vi "SaveTrendData.vi"(6 "registry":T13, 8 "error in (no error)":errorcluster, 9 "data":T9, 10 "data event config":T17, 11 "data event":T1) -> (0 "error out":errorcluster, 3 "data event out":T1)   [LabVIEW 2017, in "DataEventCreator.lvlib"]
uses:
  <vilib>/addons/InsightCM/Devices/Shared/Common/DataEventCreator/DataEventCreator.lvlib
  <vilib>/addons/InsightCM/Devices/Shared/Cms/CmsDataEventCreator/controls/DataEventConfig.ctl
  <vilib>/addons/InsightCM/Devices/Shared/Cms/CmsDataEventCreator/controls/AcqParams.ctl
  <vilib>/addons/InsightCM/Devices/Shared/Common/DataAccumulator/controls/AccumulationSettings.ctl
  <vilib>/addons/InsightCM/Devices/Shared/Common/DataAccumulator/controls/accumulationType.ctl
  <vilib>/addons/InsightCM/Devices/Shared/Common/DVRBuffer/controls/BufferLocation.ctl
  <vilib>/addons/PointValueMap/controls/PointMap.ctl
  <vilib>/addons/InsightCM/Devices/Shared/Cms/CmsDataEventCreator/controls/GroupRegistry.ctl
  <vilib>/addons/InsightCM/Devices/Shared/Cms/CmsDataEventCreator/controls/DataSetRegistry.ctl
  <vilib>/addons/InsightCM/Devices/Shared/Common/DataEvent/controls/DataSetType.ctl
  <vilib>/addons/InsightCM/Devices/Shared/Common/DataEventCreator/controls/Registry_Trend.ctl
  <vilib>/addons/InsightCM/Devices/Shared/Common/DataFlow/controls/Data.ctl
  <vilib>/addons/InsightCM/Utilities/DataAccessors/controls/wfmSGL_DVR.ctl
  <vilib>/addons/InsightCM/Devices/Shared/Common/DataFlow/controls/Type.ctl
  <vilib>/addons/InsightCM/Devices/Shared/Common/DataEvent/controls/Event.ctl
  <vilib>/addons/InsightCM/MessageBus/Base/controls/DataEvent.ctl
  <vilib>/addons/InsightCM/MessageBus/Base/controls/KeyValuePair.ctl
  <vilib>/addons/InsightCM/Devices/Shared/Common/DataEvent/controls/DataSet.ctl
  <vilib>/addons/InsightCM/MessageBus/Base/controls/DataSetMetadata.ctl
  <vilib>/addons/InsightCM/MessageBus/Base/controls/TrendPoint.ctl
  <vilib>/addons/InsightCM/MessageBus/Base/controls/TrendAlarmUpdate.ctl
  <vilib>/addons/InsightCM/MessageBus/Base/controls/TrendAlarmTransition.ctl
  <vilib>/addons/PointValueMap/subVIs/Point_Read_double.vi
  <vilib>/addons/PointValueMap/PointValueMap.lvlib
  <vilib>/addons/InsightCM/Devices/Shared/Common/DataFlow/DataFlow.lvlib
  <vilib>/addons/InsightCM/Devices/Shared/Common/DataEvent/DataEvent.lvlib
  <vilib>/addons/InsightCM/Devices/Shared/Cms/CmsDataEventCreator/CmsDataEventCreator.lvlib
  <vilib>/addons/InsightCM/Devices/Shared/Common/DataAccumulator/DataAccumulator.lvlib
  <vilib>/addons/InsightCM/Devices/Shared/Common/DVRBuffer/DVRBuffer.lvlib
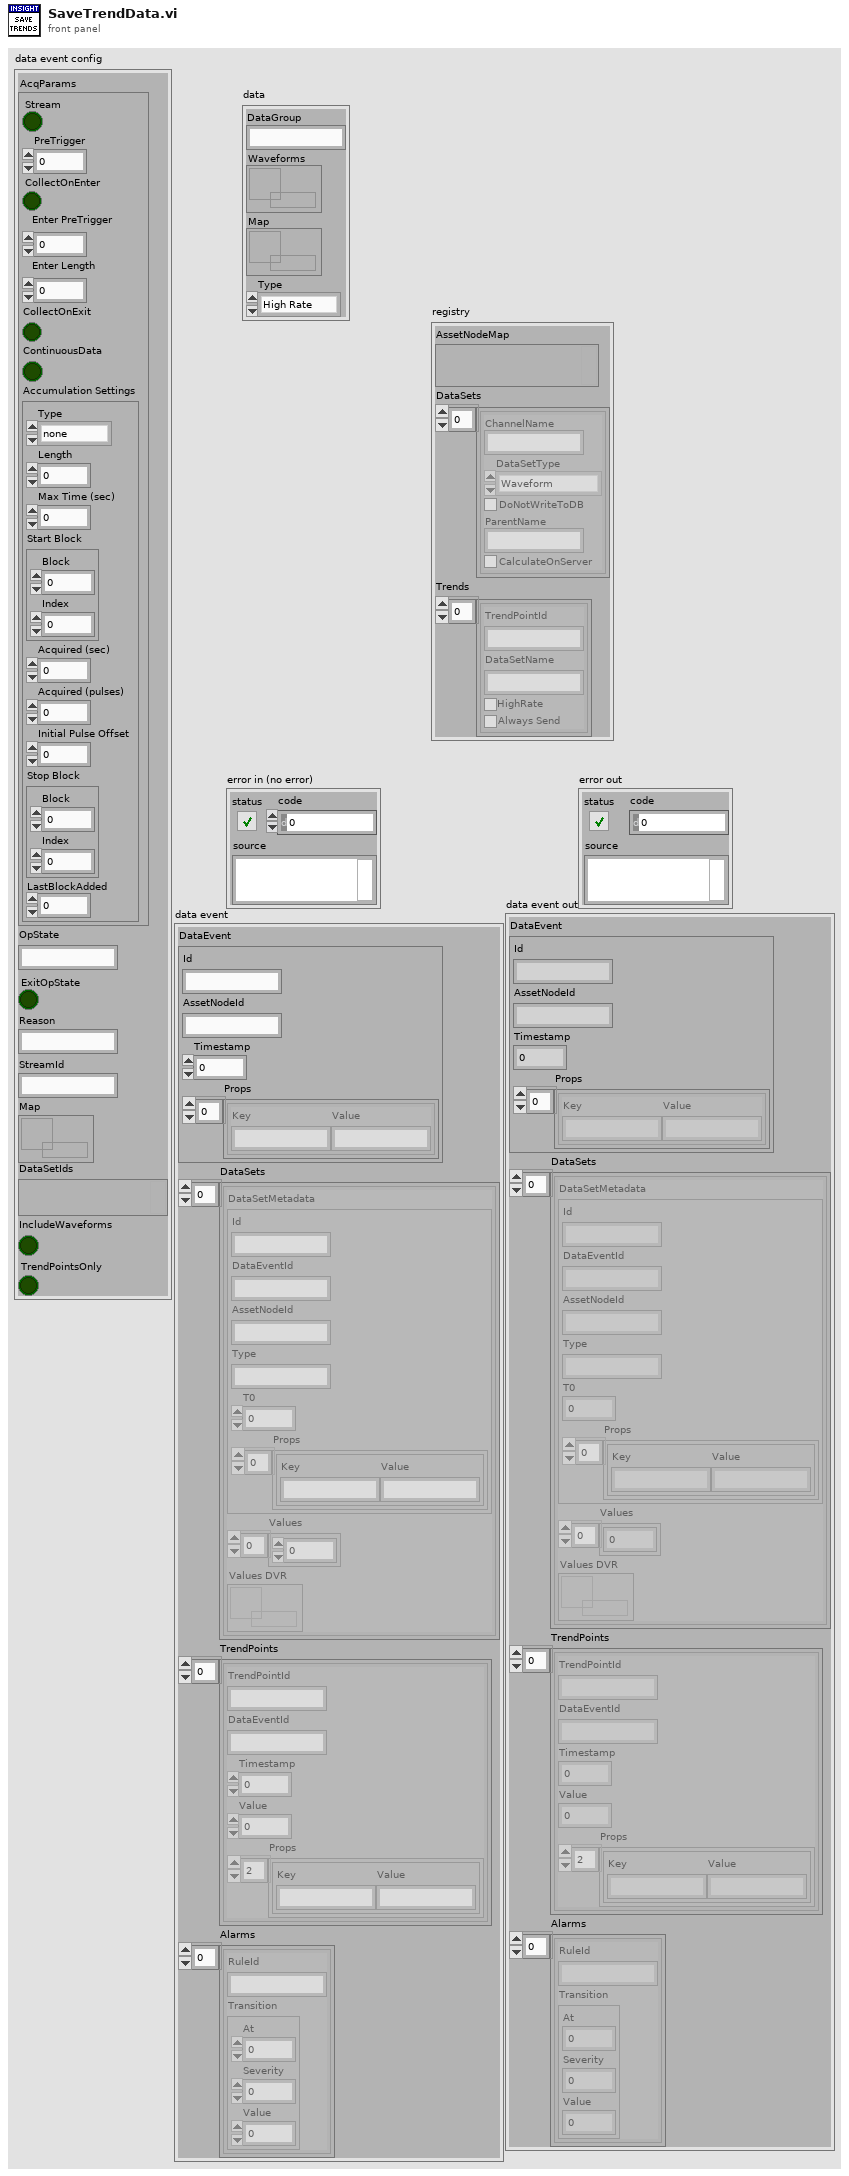
[diagram p1: front panel]
types:
  T1 = typedef "DataEvent.lvlib/Event.ctl" = cluster{"DataEvent":T2, "DataSets":T4[], "TrendPoints":T6[], "Alarms":T7[]}
  T2 = typedef "DataEvent.ctl" = cluster{"Id":string, "AssetNodeId":string, "Timestamp":i64, "Props":T3[]}
  T3 = typedef "KeyValuePair.ctl" = cluster{"Key":string, "Value":string}
  T4 = typedef "DataEvent.lvlib/DataSet.ctl" = cluster{"DataSetMetadata":T5, "Values":sgl[], "Values DVR":refnum<data-value>}
  T5 = typedef "DataSetMetadata.ctl" = cluster{"Id":string, "DataEventId":string, "AssetNodeId":string, "Type":string, "T0":i64, "Props":T3[]}
  T6 = typedef "TrendPoint.ctl" = cluster{"TrendPointId":string, "DataEventId":string, "Timestamp":i64, "Value":dbl, "Props":T3[]}
  T7 = typedef "TrendAlarmUpdate.ctl" = cluster{"RuleId":string, "Transition":T8}
  T8 = typedef "TrendAlarmTransition.ctl" = cluster{"At":i64, "Severity":i32, "Value":dbl}
  T9 = typedef "DataFlow.lvlib/Data.ctl" = cluster{"DataGroup":string, "Waveforms":T10, "Map":T11, "Type":T12}
  T10 = typedef "wfmSGL_DVR.ctl" = refnum<data-value>
  T11 = typedef "PointValueMap.lvlib/PointMap.ctl" = refnum<data-value>
  T12 = typedef "DataFlow.lvlib/Type.ctl" = enum16{"High Rate", "Low Rate", "Burst Mode"}
  T13 = typedef "CmsDataEventCreator.lvlib/GroupRegistry.ctl" = cluster{"AssetNodeMap":variant, "DataSets":T14[], "Trends":T16[]}
  T14 = typedef "CmsDataEventCreator.lvlib/DataSetRegistry.ctl" = cluster{"ChannelName":string, "DataSetType":T15, "DoNotWriteToDB":bool, "ParentName":string, "CalculateOnServer":bool}
  T15 = typedef "DataEvent.lvlib/DataSetType.ctl" = enum16{"Waveform", "SpeedProfile", "ThermalImage", "EmsaSweep"}
  T16 = typedef "DataEventCreator.lvlib/Registry_Trend.ctl" = cluster{"TrendPointId":string, "DataSetName":string, "HighRate":bool, "Always Send":bool}
  T17 = typedef "CmsDataEventCreator.lvlib/DataEventConfig.ctl" = cluster{"AcqParams":T18, "OpState":string, "ExitOpState":bool, "Reason":string, "StreamId":string, "Map":T11, "DataSetIds":variant, "IncludeWaveforms":bool, "TrendPointsOnly":bool}
  T18 = typedef "CmsDataEventCreator.lvlib/AcqParams.ctl" = cluster{"Stream":bool, "PreTrigger":i32, "CollectOnEnter":bool, "Enter PreTrigger":i32, "Enter Length":dbl, "CollectOnExit":bool, "ContinuousData":bool, "Accumulation Settings":T19}
  T19 = typedef "DataAccumulator.lvlib/AccumulationSettings.ctl" = cluster{"Type":T20, "Length":dbl, "Max Time (sec)":dbl, "Start Block":T21, "Acquired (sec)":dbl, "Acquired (pulses)":i32, "Initial Pulse Offset":dbl, "Stop Block":T21, "LastBlockAdded":u32}
  T20 = typedef "DataAccumulator.lvlib/accumulationType.ctl" = enum16{"none", "seconds", "revolutions"}
  T21 = typedef "DVRBuffer.lvlib/BufferLocation.ctl" = cluster{"Block":u32, "Index":i32}
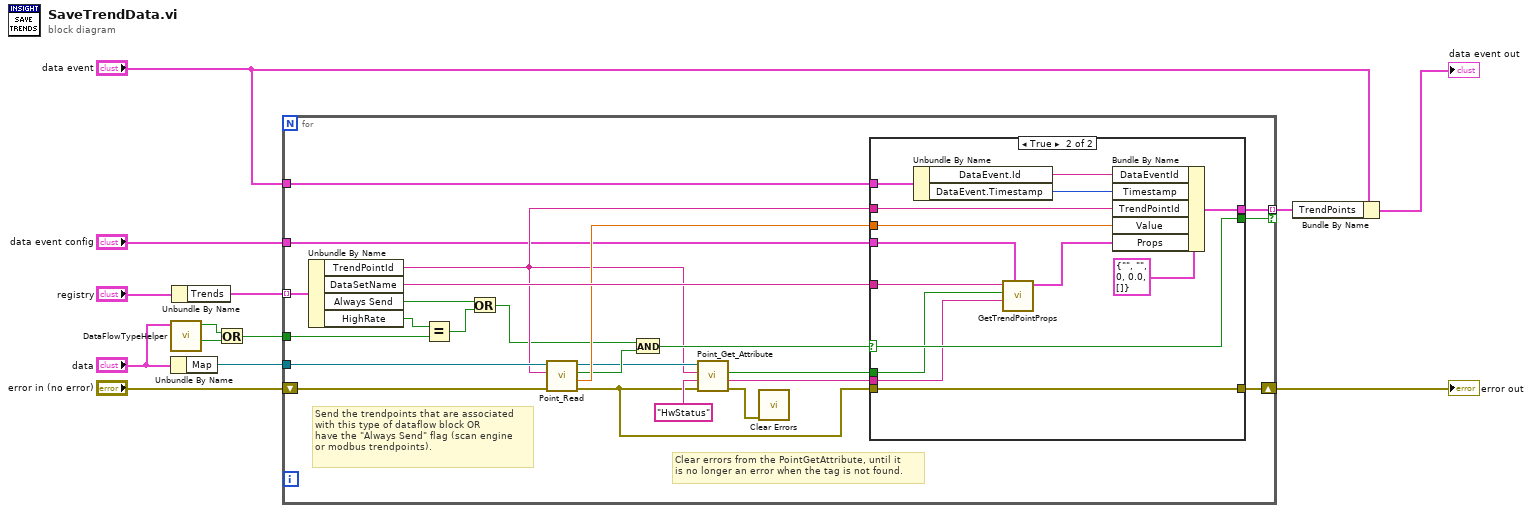
[diagram p0: block diagram]
diagram:
  n1 = call <vilib>:"DataFlowTypeHelper.vi"("data"="data") -> ("burst mode"=w3:bool, "high rate"=w2:bool)  [unwired: 8 in, 1 out]
  n2 = Unbundle By Name("data") -> ("Map"=w9:T11)
  n3 = Unbundle By Name("registry") -> ("Trends"=w10:T16[])
  n4 = Or(x=w2, y=w3) -> (x .or. y?=w1:bool)
  n5 = for {
    tunnel: w9 -> [w35]
    tunnel: w10 -> [w34] mode=indexing
    shift-right: [w23] -> w12
    shift-left: "error in (no error)" -> [w36]
    tunnel: "data event" -> [w33]
    tunnel: [w32] -> w6 mode=indexing if=w30
    tunnel: w1 -> [w29]
    tunnel: "data event config" -> [w20]
    # "Clear errors from the PointGetAttribute, until it \nis no longer an error when the tag is not found."
    # "Send the trendpoints that are associated\nwith this type of dataflow block OR\nhave the \"Always Send\" flag (scan engine\nor modbus trendpoints)."
    n6 = Unbundle By Name(w34) -> ("TrendPointId"=w25:string, "DataSetName"=w37:string, "Always Send"=w16:bool, "HighRate"=w17:bool)
    n7 = Equal?(x=w17, y=w29) -> (x = y?=w15:bool)
    n8 = Or(x=w16, y=w15) -> (x .or. y?=w14:bool)
    n9 = call-poly <vilib>:"Point_Read.vi"("Error In"=w36, "Tag"=w25, "Map"=w35) -> ("Error Out"=w18:errorcluster, "Value"=w31:dbl, "Found?"=w28:bool, "Map Out"=w26:T11)  [unwired: 3 in, 2 out]
    n10 = And(x=w14, y=w28) -> (x .and. y?=w27:bool)
    n11 = call <vilib>:"Point_Get_Attribute.vi"("Error In"=w18, "Attribute"="HwStatus", "Tag"=w25, "Map"=w26) -> ("Error Out"=w19:errorcluster, "Value"=w21:string, "Found?"=w22:bool)  [unwired: 4 in, 1 out]
    n12 = call <vilib>:"Clear Errors.vi"("error in (no error)"=w19) -> ()  [unwired: 5 in, 2 out]
    n13 = case shown="True" w27 {
      selector: w27 -> [w39 w44]
      tunnel: w37 -> [_ w53]
      tunnel: w33 -> [_ w52]
      tunnel: [_ w48] -> w32
      tunnel: w31 -> [_ w47]
      tunnel: w25 -> [_ w45]
      tunnel: [w39 w44] -> w30
      tunnel: [w38 w43] -> w23
      tunnel: w18 -> [w38 w43]
      tunnel: w22 -> [_ w42]
      tunnel: w21 -> [_ w40]
      tunnel: w20 -> [_ w41]
      frame False {
      }
      frame True {
        n14 = Unbundle By Name(w52) -> ("DataEvent.Id"=w50:string, "DataEvent.Timestamp"=w49:i64)
        n15 = call <vilib>:"GetTrendPointProps.vi"("data event"=w41, "hw status"=w40, "found hw status"=w42, "DataSetName"=w53) -> ("key value pairs out"=w46:T3[])  [unwired: 7 in]
        n16 = Bundle By Name(cluster=T6 {"TrendPointId"="", "DataEventId"="", "Timestamp"=0, "Value"=0.0, "Props"=[]} ("TrendPoint"), "DataEventId"=w50, "Timestamp"=w49, "TrendPointId"=w45, "Value"=w47, "Props"=w46) -> (w48:T6)
      }
    }
  }
  "error out" <- w12
  n17 = Bundle By Name(cluster="data event", "TrendPoints"=w6) -> (→"data event out":T1)
